vi "Claw Position Activate.vi"(9 "Claw Retract":bool, 11 "Claw Extend":bool) -> ()   [LabVIEW 2012]
uses:
  <vilib>/Rock Robotics/WPI/Solenoid/WPI_SolenoidValue.ctl
  <vilib>/Rock Robotics/WPI/Solenoid/WPI_SolenoidSetEnum.vi
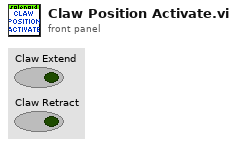
[diagram p1: front panel]
types:
  T1 = typedef "WPI_SolenoidValue.ctl" = enum16{"Off", "On", "Forward", "Reverse"}
  T2 = typedef "WPI_SolenoidDevRef.ctl" = cluster{"DevStatus":errorcluster, "Solenoid Module":T3, "Forward Solenoid Channel":T4, "Reverse Solenoid Channel":T4}
  T3 = typedef "FPGA_TypedefSolenoidModule.ctl" = enum16{"Solenoid Module 1", "Solenoid Module 2"}
  T4 = typedef "WPI_SolenoidChannel.ctl" = enum8{"Solenoid 1", "Solenoid 2", "Solenoid 3", "Solenoid 4", "Solenoid 5", "Solenoid 6", "Solenoid 7", "Solenoid 8", "Invalid"}
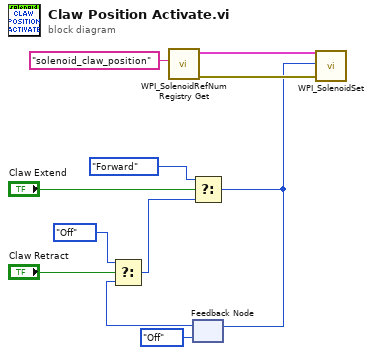
[diagram p0: block diagram]
diagram:
  n1 = call <vilib>:"WPI_SolenoidRefNum Registry Get.vi"("refnum name"="solenoid_claw_position") -> ("error out"=w10:errorcluster, "SolenoidDevRef"=w11:T2)  [unwired: 9 in]
  n2 = feedback #1(WPI_SolenoidValue."Off" ("Value")) -> (w2:T1)
  n3 = Select(t=WPI_SolenoidValue."Off" ("Value"), s="Claw Retract", f=w2) -> (s? t:f=w4:T1)
  n4 = Select(t=WPI_SolenoidValue."Forward" ("Value"), s="Claw Extend", f=w4) -> (s? t:f=w3:T1)
  n5 = feedback-in #1(w3) -> ()
  n6 = call-poly <vilib>:"WPI_SolenoidSet.vi"("error in (no error)"=w10, "Value"=w3, "SolenoidDevRef"=w11) -> ()  [unwired: 7 in, 2 out]
